vi "EventClient_Destroy.vi"(8 "error in (no error)":errorcluster, 11 "reference":T1) -> (0 "error out":errorcluster)   [LabVIEW 2011]
uses:
  EventClient_ObjectReference.ctl
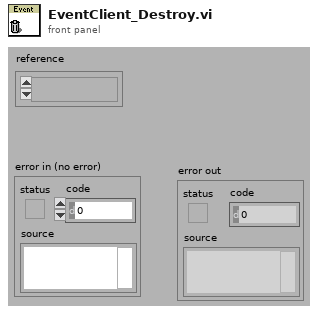
[diagram p1: front panel]
types:
  T1 = typedef "EventClient_ObjectReference.ctl" = refnum<k1>
  T2 = cluster{"Client":refnum<queue>, "Sub Events":string[], "PrvData":variant, "MyName":string}
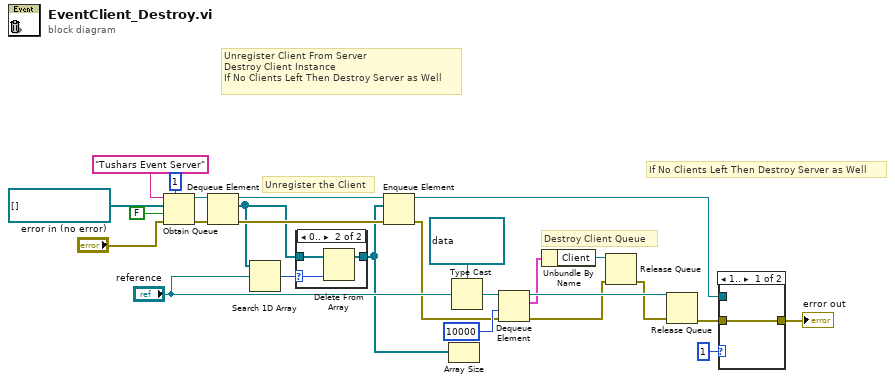
[diagram p0: block diagram]
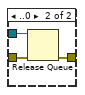
[diagram p2: hidden frame]
diagram:
  w19 = T1[] [] items=["EventClient"]
  # "If No Clients Left Then Destroy Server as Well"
  # "Unregister Client From Server\nDestroy Client Instance\nIf No Clients Left Then Destroy Server as Well"
  # "Destroy Client Queue"
  # "Unregister the Client"
  n1 = Obtain Queue(max queue size (-1, unlimited)=1, name (unnamed)="Tushars Event Server", element data type=w19, create if not found? (T)=FALSE, error in (no error)="error in (no error)") -> (queue out=w21:refnum<queue>, error out=w22:errorcluster)  [unwired: 1 out]
  n2 = Dequeue Element(queue=w21, error in (no error)=w22) -> (queue out=w15:refnum<queue>, element=w12:T1[], error out=w14:errorcluster)  [unwired: 2 out]
  n3 = Search 1D Array(1D array=w12, element="reference") -> (index of element=w13:i32)  [unwired: 1 out]
  n4 = case shown="0.." w13 {
    selector: w13 -> [_ w28]
    tunnel: w12 -> [w27 w30]
    tunnel: [w27 w29] -> w7
    frame ..-1 {
    }
    frame 0.. {
      n5 = Delete From Array(array=w30, index=w28) -> (array with subset deleted=w29:T1[])  [unwired: 1 in, 1 out]
    }
  }
  n6 = Enqueue Element(queue=w15, element=w7, error in (no error)=w14) -> (queue out=w4:refnum<queue>, error out=w16:errorcluster)  [unwired: 2 out]
  n7 = Array Size(array=w7) -> ()  [unwired: 1 out]
  n8 = Type Cast(type=refnum<queue> refnum ("queue out"), x="reference") -> (*(type *) &x=w24:refnum<queue>)
  n9 = Dequeue Element(queue=w24, timeout in ms (-1)=10000 ("timeout in ms (10000)"), error in (no error)=w16) -> (queue out=w25:refnum<queue>, element=w11:T2, error out=w9:errorcluster)  [unwired: 1 out]
  n10 = Unbundle By Name(w11) -> ("Client"=w10:refnum<queue>)
  n11 = Release Queue(queue=w10, error in (no error)=w9) -> (error out=w8:errorcluster)  [unwired: 3 out]
  n12 = Release Queue(queue=w25, error in (no error)=w8) -> (error out=w6:errorcluster)  [unwired: 3 out]
  n13 = case shown="1.." 1 {
    tunnel: w6 -> [w31 w34]
    tunnel: [w31 w33] -> w5
    tunnel: w4 -> [_ w32]
    frame 1.. {
    }
    frame ..0 {
      n14 = Release Queue(queue=w32, error in (no error)=w34) -> (error out=w33:errorcluster)  [unwired: 3 out]
    }
  }
  "error out" <- w5
